vi "Decode Reg Number.vi"(4 "String":string="218004116") -> (0 "Reg Number":i32, 1 "Campus":string="218004116", 2 "Department":string="218004116", 3 "Year":string)   [LabVIEW 2014]
panel:
  out "substring":string
  out "date string":string
  out "Campus":u8
  out "Year of Passing":i32
  out "Department":i8
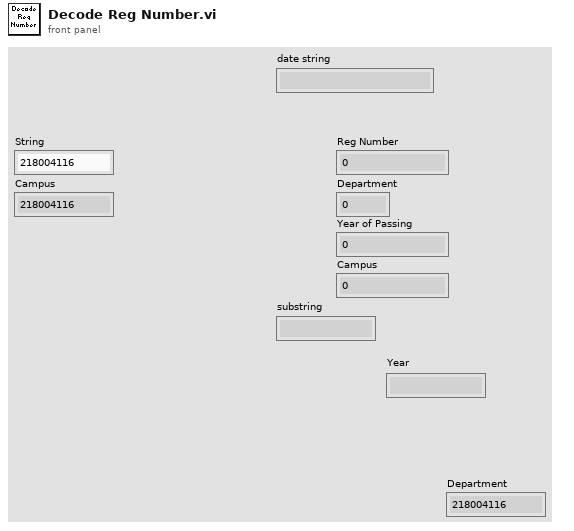
[diagram p1: front panel]
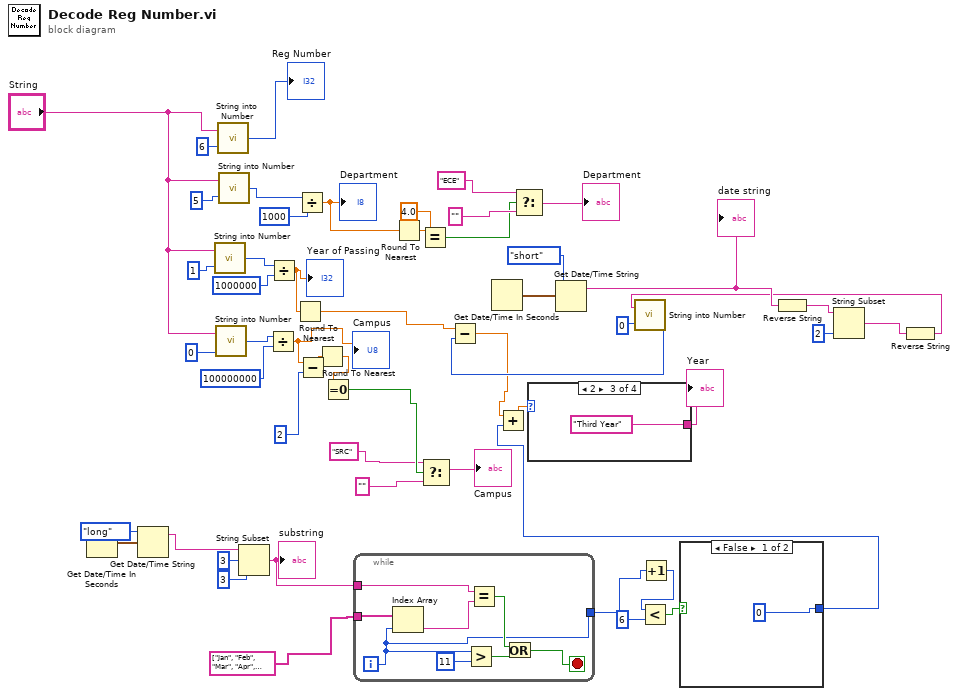
[diagram p0: block diagram]
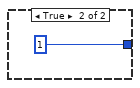
[diagram p2: hidden frame]
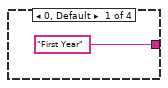
[diagram p3: hidden frame]
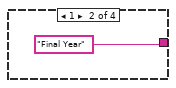
[diagram p4: hidden frame]
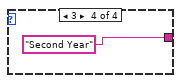
[diagram p5: hidden frame]
diagram:
  n1 = Get Date/Time In Seconds() -> (seconds since 1Jan1904=w3:timestamp)
  n2 = Get Date/Time String(date format (0)=enum16{"short", "long", "abbreviated"}."long", seconds (now)=w3) -> (date string=w2:string)  [unwired: 1 in, 1 out]
  n3 = call "String into Number.vi"("initial scan location"=u32 1, "String"="String") -> ("output 1"=w48:i32)
  n4 = call "String into Number.vi"("initial scan location"=u32 0, "String"="String") -> ("output 1"=w44:i32)
  n5 = call "String into Number.vi"("initial scan location"=u32 6, "String"="String") -> ("output 1"=→"Reg Number":i32)
  n6 = call "String into Number.vi"("initial scan location"=u32 5, "String"="String") -> ("output 1"=w49:i32)
  n7 = String Subset(string=w2, offset (0)=3, length (rest)=3 ("length (rest)")) -> (substring=w16:string)
  "substring" <- w16
  n8 = Divide(x=w44, y=100000000) -> (x/y=w39:dbl)
  "Campus" <- w39
  n9 = Divide(x=w48, y=1000000) -> (x/y=w31:dbl)
  "Year of Passing" <- w31
  n10 = Round To Nearest(number=w31) -> (nearest integer value=w30:dbl)
  n11 = Divide(x=w49, y=1000) -> (x/y=w29:dbl)
  "Department" <- w29
  n12 = Subtract(x=w39, y=u32 2 ("initial scan location")) -> (x-y=w36:dbl)
  n13 = Round To Nearest(number=w36) -> (nearest integer value=w37:dbl)
  n14 = Equal To 0?(x=w37) -> (x = 0?=w32:bool)
  n15 = while {
    tunnel: string[] ["Jan", "Feb", "Mar", "Apr", "May", "Jun", "Jul", "Aug", "Sep", "Oct", "Nov", "Dec"] ("Array") -> [w61]
    tunnel: w16 -> [w59]
    tunnel: [w54] -> w15
    i -> [w54]
    stop <- w58 stop-if-true
    n16 = Index Array(array=w61, index=w54) -> (element=w60:string)
    n17 = Greater?(x=w54, y=11) -> (0:w56:bool)
    n18 = Equal?(x=w59, y=w60) -> (x = y?=w57:bool)
    n19 = Or(x=w57, y=w56) -> (x .or. y?=w58:bool)
  }
  n20 = Round To Nearest(number=w29) -> (nearest integer value=w28:dbl)
  n21 = Equal?(x=w28, y=4.0) -> (x = y?=w26:bool)
  n22 = Select(t="SRC" ("String 2"), s=w32, f="" ("String 2")) -> (s? t:f=→"Campus":string)
  n23 = Get Date/Time In Seconds() -> (seconds since 1Jan1904=w23:timestamp)
  n24 = Select(t="ECE" ("String 2"), s=w26, f="" ("String 2")) -> (s? t:f=→"Department":string)
  n25 = Get Date/Time String(date format (0)=enum16{"short", "long", "abbreviated"}."short", seconds (now)=w23) -> (date string=w8:string)  [unwired: 1 in, 1 out]
  "date string" <- w8
  n26 = Increment(x=w15) -> (x+1=w13:i32)
  n27 = Less?(x=w13, y=6) -> (x < y?=w14:bool)
  n28 = case shown="False" w14 {
    tunnel: [0 ("y") 1 ("y")] -> w9
    frame False {
    }
    frame True {
    }
  }
  n29 = Reverse String(1:w8) -> (0:w7:string)
  n30 = String Subset(string=w7, length (rest)=2 ("length (rest)")) -> (substring=w5:string)  [unwired: 1 in]
  n31 = Reverse String(1:w5) -> (0:w4:string)
  n32 = call "String into Number.vi"("initial scan location"=u32 0, "String"=w4) -> ("output 1"=w22:i32)
  n33 = Subtract(x=w30, y=w22) -> (x-y=w10:dbl)
  n34 = Add(x=w10, y=w9) -> (x+y=w11:dbl)
  n35 = case shown="2" w11 {
    tunnel: ["First Year" ("String 2") "Final Year" ("String 2") "Third Year" ("String 2") "Second Year" ("String 2")] -> w21
    frame 0, Default {
    }
    frame 1 {
    }
    frame 2 {
    }
    frame 3 {
    }
  }
  "Year" <- w21
